vi "Constructor.vi"(8 "error in (no error)":errorcluster, 11 "Ethernet MAC - Custom in":refnum<class "Ethernet MAC - Custom.lvclass">) -> (0 "error out":errorcluster, 3 "Ethernet MAC - Custom out":refnum<class "Ethernet MAC - Custom.lvclass">)   [LabVIEW 2020]
uses:
  Ethernet MAC - Custom.lvclass
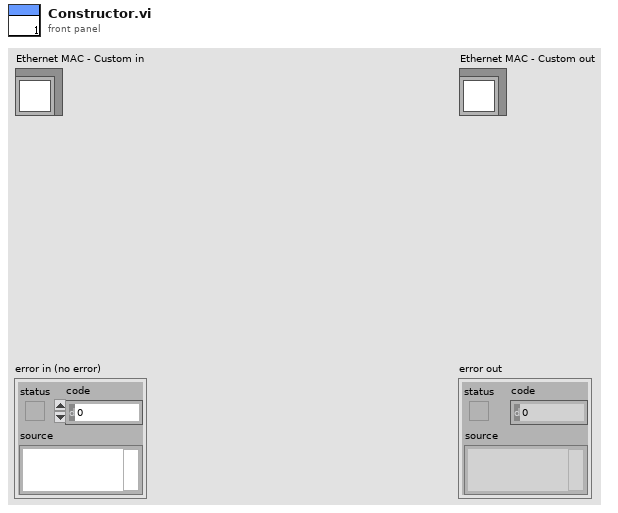
[diagram p1: front panel]
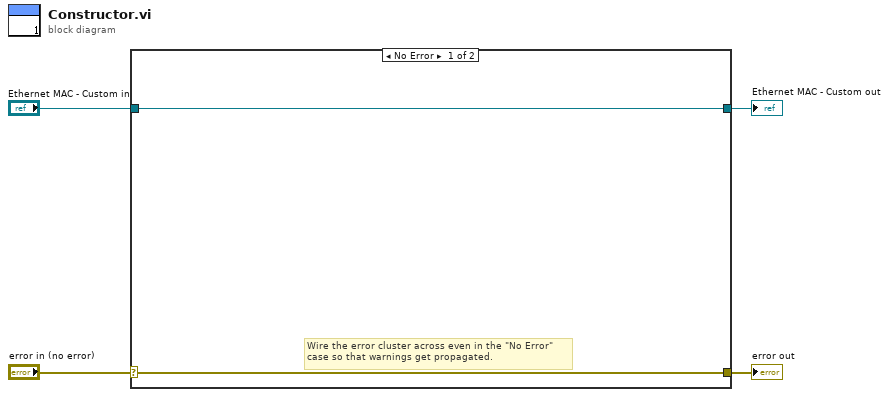
[diagram p0: block diagram]
diagram:
  n1 = case shown="No Error" "error in (no error)" {
    selector: "error in (no error)" -> [w5 w8]
    tunnel: [w5 w8] -> w3
    tunnel: [w6 w7] -> w1
    tunnel: "Ethernet MAC - Custom in" -> [w6 w7]
    frame No Error {
      # "Wire the error cluster across even in the \"No Error\"\ncase so that warnings get propagated."
    }
    frame Error {
    }
  }
  "error out" <- w3
  "Ethernet MAC - Custom out" <- w1
